vi "header_spectrum_sheet.vi"(1 "WAVELENGTH":dbl[](array[numeric])) -> (0 "chaîne concaténée":string)   [LabVIEW 2018]
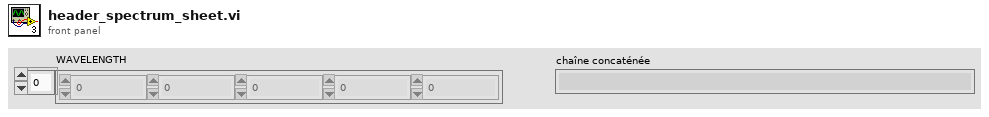
[diagram p1: front panel]
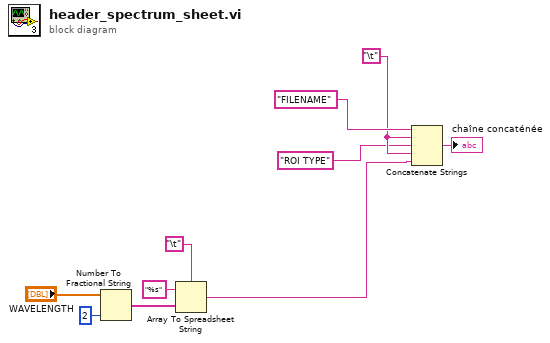
[diagram p0: block diagram]
diagram:
  w6 = "\t"
  n1 = Number To Fractional String(number="WAVELENGTH", precision (6)=i16 2 ("précision (6)")) -> (F-format string=w8:string[])  [unwired: 2 in]
  n2 = Array To Spreadsheet String(delimiter (Tab)="\t", array=w8, 3:"%s" ("chaîne de format")) -> (spreadsheet string=w4:string)
  n3 = Concatenate Strings("FILENAME", w6, "ROI TYPE", w6, w4) -> (→"chaîne concaténée":string)
